vi "Configure Control Output.vi"(0 "VISA resource name":refnum<visa-resource-name>, 1 "Control Output (0: 1A)":i16(ring) items=["1A", "1B", "2A", "2B"], 2 "Process Output Type (0: 4 to 20 mA)":u16(ring) items=["4 to 20 mA", "0 to 20 mA", "0 to 5 V", "1 to 5 V", "0 to 10 V"], 3 "High Power Limit (100.0)":dbl=100.0 format="%.2f", 4 "Low Power Limit (0.0)":dbl format="%.2f", 5 "error in (no error)":errorcluster {"code" format="%.0x"}, 6 "Unit Address (1)":i16=1, 8 "Function (1: Heat)":u16(ring)=1 items=["Off", "Heat", "Cool"], 10 "Choose Cycle Time (1: Fixed Time)":u16(ring)=1 items=["Variable Burst", "Fixed Time"], 12 "Enter Cycle Time (1.0)":dbl=1.0 format="%.2f") -> (14 "VISA resource name out":refnum<visa-resource-name>, 19 "error out":errorcluster {"code" format="%.0x"})   [LabVIEW 2010]
doc: "This VI configures control outputs."
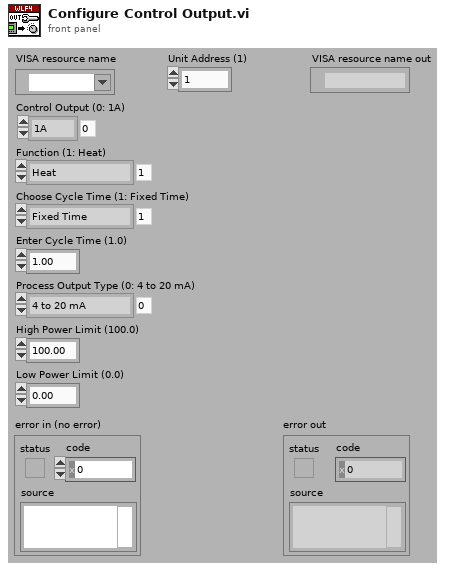
[diagram p1: front panel]
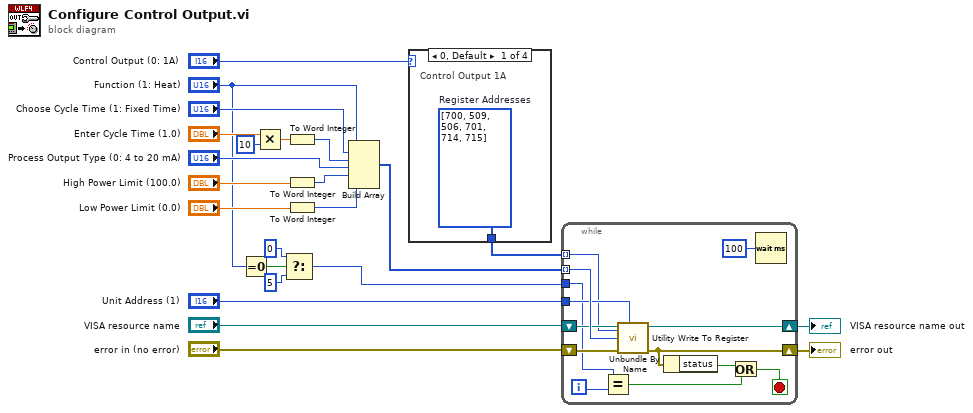
[diagram p0: block diagram]
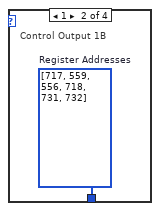
[diagram p2: hidden frame]
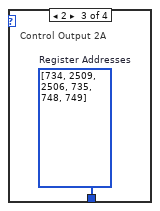
[diagram p3: hidden frame]
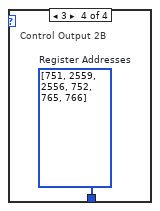
[diagram p4: hidden frame]
diagram:
  n1 = Equal To 0?(x="Function (1: Heat)") -> (x = 0?=w5:bool)
  n2 = Multiply(x="Enter Cycle Time (1.0)", y=i16 10) -> (x*y=w14:dbl)
  n3 = Select(t=i16 0, s=w5, f=i16 5 ("t")) -> (s? t:f=w1:i16)
  n4 = To Word Integer(number=w14) -> (16bit integer=w15:i16)
  n5 = To Word Integer(number="High Power Limit (100.0)") -> (16bit integer=w8:i16)
  n6 = To Word Integer(number="Low Power Limit (0.0)") -> (16bit integer=w7:i16)
  n7 = Build Array("Function (1: Heat)", "Choose Cycle Time (1: Fixed Time)", w15, "Process Output Type (0: 4 to 20 mA)", w8, w7) -> (w18:u16[])
  n8 = case shown="0, Default" "Control Output (0: 1A)" {
    tunnel: [w24 w25 w26 w27] -> w17
    frame 0, Default {
      w24 = i32[] [700, 509, 506, 701, 714, 715]  # Register Addresses
      # "Control Output 1A"
    }
    frame 1 {
      w25 = i32[] [717, 559, 556, 718, 731, 732]  # Register Addresses
      # "Control Output 1B"
    }
    frame 2 {
      w26 = i32[] [734, 2509, 2506, 735, 748, 749]  # Register Addresses
      # "Control Output 2A"
    }
    frame 3 {
      w27 = i32[] [751, 2559, 2556, 752, 765, 766]  # Register Addresses
      # "Control Output 2B"
    }
  }
  n9 = while {
    tunnel: w18 -> [w40] mode=indexing
    tunnel: "Unit Address (1)" -> [w39]
    shift-right: [w36] -> w21
    shift-left: "VISA resource name" -> [w38]
    shift-right: [w33] -> w20
    shift-left: "error in (no error)" -> [w37]
    tunnel: w17 -> [w34] mode=indexing
    tunnel: w1 -> [w28]
    i -> [w30]
    stop <- w31 stop-if-true
    n10 = Equal?(x=w28, y=w30) -> (x = y?=w29:bool)
    n11 = call "Utility Write To Register.vi"("Unit Address (1)"=w39, "error in (no error)"=w37, "Data (0)"=w40, "Register Address (0)"=w34, "VISA resource name"=w38) -> ("error out"=w33:errorcluster, "VISA resource name out"=w36:refnum<visa-resource-name>)  [unwired: 5 in]
    n12 = Unbundle By Name(w33) -> ("status"=w32:bool)
    n13 = Or(x=w32, y=w29) -> (x .or. y?=w31:bool)
    n14 = Wait (ms)(milliseconds to wait=u32 100) -> ()  [unwired: 1 out]
  }
  "error out" <- w20
  "VISA resource name out" <- w21
